vi "Relabel It.vi"(0 "Index":i32=-2000000000, 1 "# of columns":i32=-10, 2 "Column Headings":string[](array[string])=["Field", "Voltage1", "Voltage2", "Temp", "Timestamp", "", "", "", "", "", "", "", "", "", "", "", "", "", ""], 3 "Display?":bool[](array[boolean])=[FALSE, FALSE, FALSE, FALSE, FALSE, FALSE, FALSE, FALSE, FALSE, FALSE, FALSE, FALSE, FALSE, FALSE, FALSE, FALSE, FALSE], 4 "X-Axis":i32(ring)=1 items=["Point #", "Field", "Voltage1"]) -> (5 "?":bool=TRUE)   [LabVIEW 2024]
doc: "This VI decides if there is more data or if the plot parameters have changed. If not then returns false."
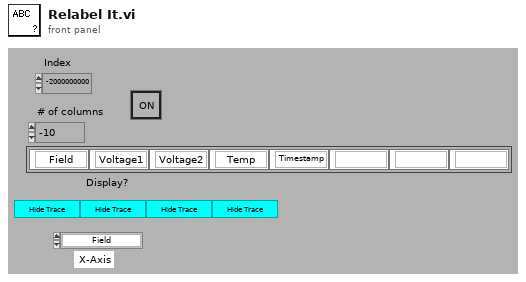
[diagram p1: front panel]
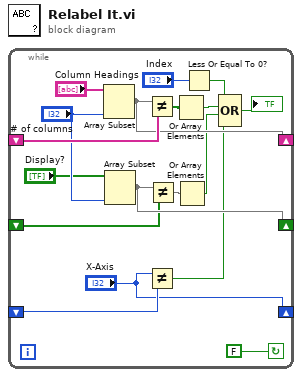
[diagram p0: block diagram]
diagram:
  n1 = while {
    shift-left: _ -> [w4]
    shift-right: ["X-Axis"] -> _
    shift-left: _ -> [w8]
    shift-right: [w9] -> _
    shift-left: _ -> [w17]
    shift-right: [w12] -> _
    stop <- FALSE continue-if-true
    n2 = Array Subset(array="Column Headings", length="# of columns") -> (w12:string[])  [unwired: 1 in]
    n3 = Array Subset(array="Display?", length="# of columns") -> (w9:bool[])  [unwired: 1 in]
    n4 = Not Equal?(x=w12, y=w17) -> (x != y?=w15:bool[])
    n5 = Not Equal?(x="X-Axis", y=w4) -> (x != y?=w2:bool)
    n6 = Not Equal?(x=w9, y=w8) -> (x != y?=w10:bool[])
    n7 = Or Array Elements(Boolean array=w15) -> (logical OR=w14:bool)
    n8 = Or Array Elements(Boolean array=w10) -> (logical OR=w5:bool)
    n9 = Less Or Equal To 0?(x="Index") -> (x <= 0?=w18:bool)
    n10 = Compound Arithmetic op=OR(w18, w14, w5, w2) -> (→"?":bool)
  }
